vi "Module.Init Working Dirs.vi"(7 "Public Docs":bool, 8 "error in":errorcluster, 11 "App Name":string) -> (0 "error out":errorcluster, 3 "Working Dirs":T1)   [LabVIEW 2024, in "EQMF.lvlib" / "Module Utils.lvlib"]
uses:
  Module Utils.lvlib
  Module.Working Dirs.ctl
  <vilib>/Utility/sysdir.llb/System Directory Type.ctl
  <vilib>/Utility/config.llb/Read Key (Path).vi
  <vilib>/Utility/config.llb/NI_LVConfig.lvlib
  Files/File Utils.lvlib
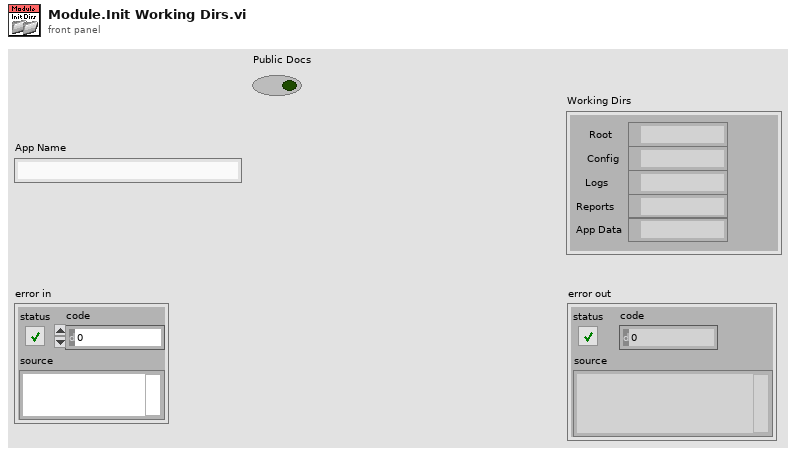
[diagram p1: front panel]
types:
  T1 = typedef "EQMF.lvlib/Module Utils.lvlib/Module.Working Dirs.ctl" = cluster{"Root":path, "Config":path, "Logs":path, "Reports":path, "App Data":path}
  T2 = enum32{"invalid app kind", "Development System", "Run Time System", "Student Edition", "Embedded LabVIEW", "Evaluation", "Custom"}
  T3 = cluster{"Working Dir":path, "Local Config File":path}
  T4 = typedef "NI_LVConfig.lvlib/Config Data RefNum.ctl" = refnum<k1>
  T5 = typedef "System Directory Type.ctl" = i32
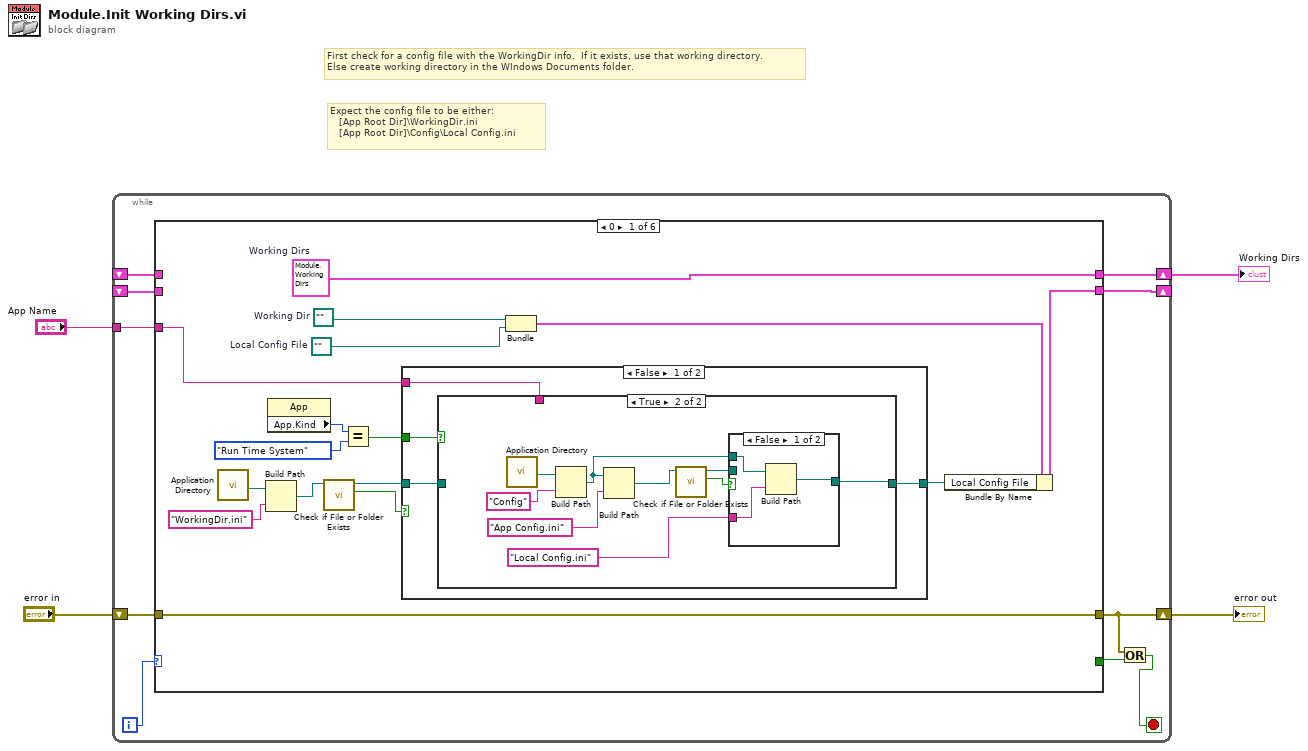
[diagram p0: block diagram]
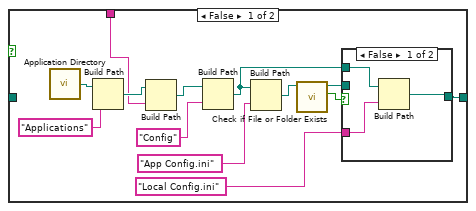
[diagram p2: hidden frame]
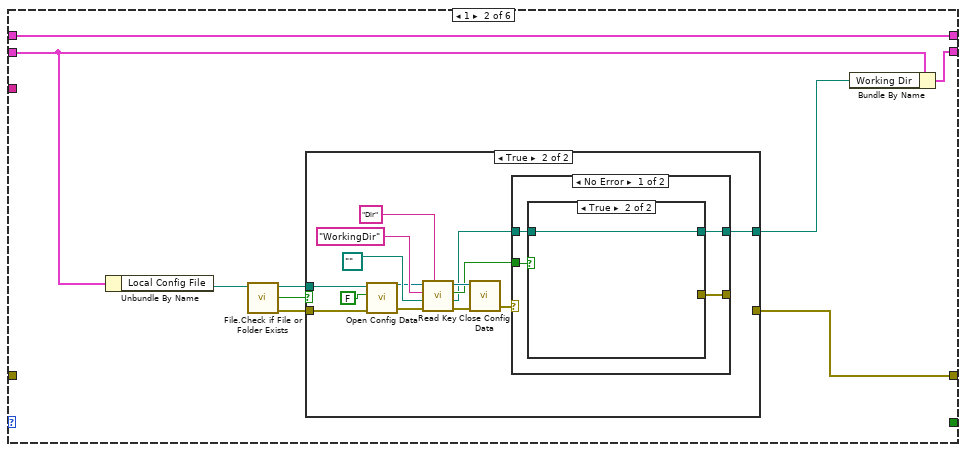
[diagram p6: hidden frame]
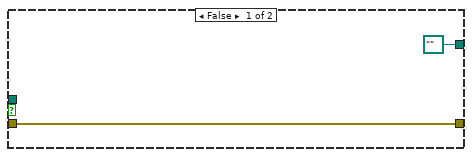
[diagram p7: hidden frame]
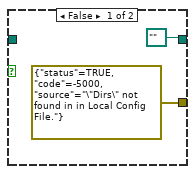
[diagram p8: hidden frame]
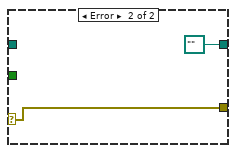
[diagram p9: hidden frame]
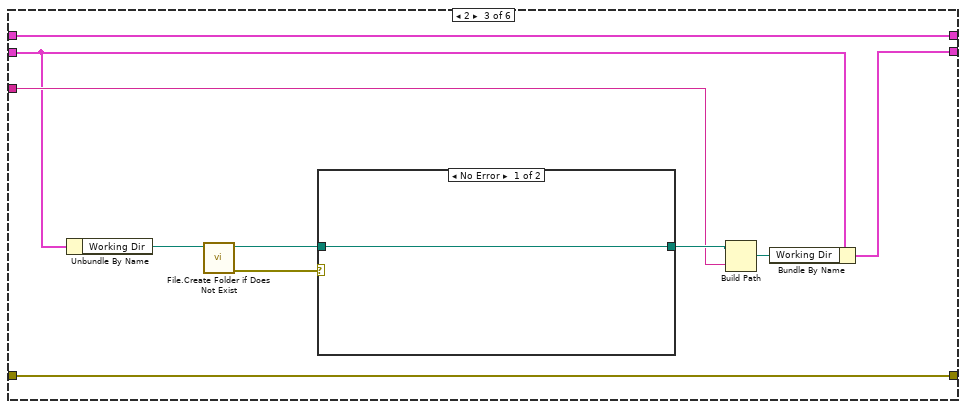
[diagram p10: hidden frame]
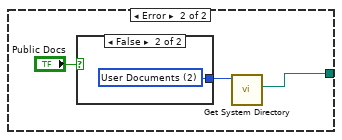
[diagram p11: hidden frame]
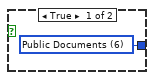
[diagram p12: hidden frame]
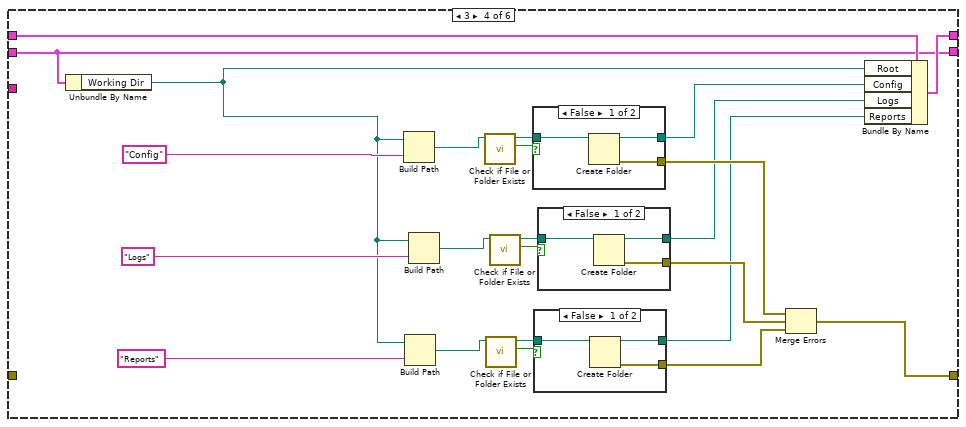
[diagram p13: hidden frame]
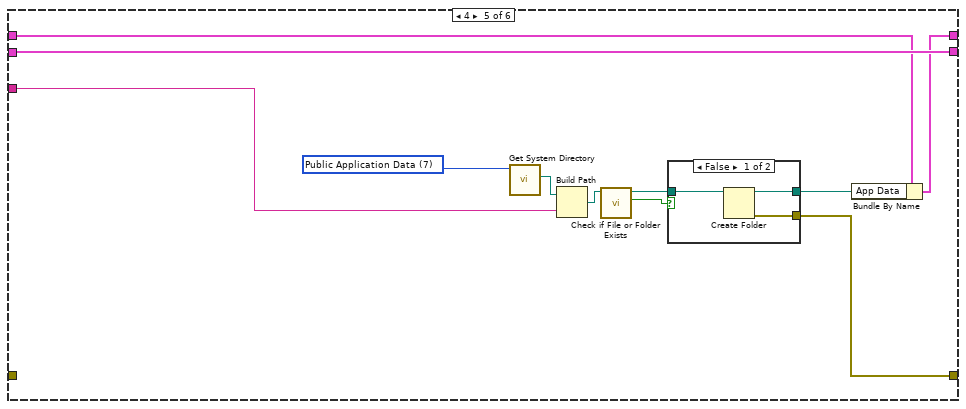
[diagram p17: hidden frame]
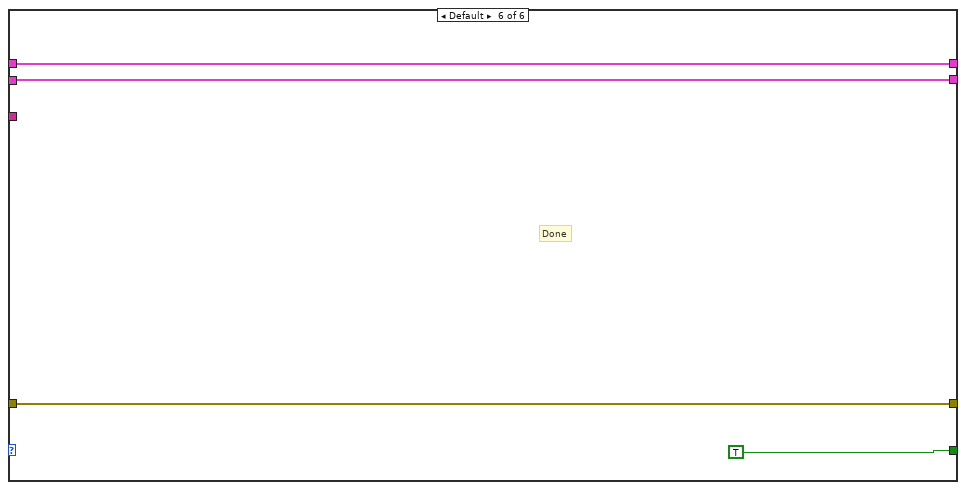
[diagram p19: hidden frame]
diagram:
  # "Expect the config file to be either:\n   [App Root Dir]\\WorkingDir.ini\n   [App Root Dir]\\Config\\Local Config.ini"
  # "First check for a config file with the WorkingDir info.  If it exists, use that working directory.\nElse create working directory in the WIndows Documents folder."
  n1 = while {
    shift-right: [w10] -> w3
    shift-left: "error in" -> [w13]
    shift-right: [w12] -> w1
    shift-left: _ -> [w7]
    tunnel: "App Name" -> [w8]
    shift-right: [w5] -> _
    shift-left: _ -> [w6]
    i -> [w14]
    stop <- w9 stop-if-true
    n2 = case shown="0" w14 {
      tunnel: [_ _ _ _ _ TRUE] -> w11
      tunnel: [w29 w70 w103 w118 w155 w168] -> w10
      tunnel: w13 -> [w29 _ w103 _ _ w168]
      tunnel: [w30 w71 w109 w137 w152 w167] -> w12
      tunnel: w8 -> [w16 _ w106 _ w156 _]
      tunnel: w7 -> [_ w71 w109 w138 w153 w167]
      tunnel: w6 -> [_ w68 w104 w116 w154 w166]
      tunnel: [w25 w69 w105 w116 w154 w166] -> w5
      frame 0 {
        w27 = path ""  # Local Config File
        w28 = path ""  # Working Dir
        w30 = T1 {"Root"=path "", "Config"=path "", "Logs"=path "", "Reports"=path "", "App Data"=path ""}  # Working Dirs
        n3 = call <vilib>:"Application Directory.vi"() -> ("Application Directory"=w21:path)
        n4 = Build Path(base path=w21, name or relative path="WorkingDir.ini") -> (appended path=w22:path)
        n5 = property class="App"() -> ("App.Kind"=w19:T2)  [unwired: 2 in, 2 out]
        n6 = call <vilib>:"Check if File or Folder Exists.vi"("path"=w22) -> ("file or folder exists?"=w24:bool, "dup path"=w23:path)  [unwired: 8 in, 1 out]
        n7 = Equal?(x=w19, y=T2."Run Time System" ("Application:Kind")) -> (x = y?=w20:bool)
        n8 = case shown="False" w24 {
          tunnel: w20 -> [w34 _]
          tunnel: w23 -> [w33 w65]
          tunnel: [w32 w65] -> w15
          tunnel: w16 -> [w31 _]
          frame False {
            n9 = case shown="True" w34 {
              tunnel: [w37 w53] -> w32
              tunnel: w33 -> [_ _]
              tunnel: w31 -> [w41 _]
              frame False {
                n10 = call <vilib>:"Application Directory.vi"() -> ("Application Directory"=w45:path)
                n11 = Build Path(base path=w45, name or relative path="Applications") -> (appended path=w46:path)
                n12 = Build Path(base path=w46, name or relative path=w41) -> (appended path=w47:path)
                n13 = Build Path(base path=w47, name or relative path="Config") -> (appended path=w35:path)
                n14 = Build Path(base path=w35, name or relative path="App Config.ini") -> (appended path=w40:path)
                n15 = call <vilib>:"Check if File or Folder Exists.vi"("path"=w40) -> ("file or folder exists?"=w39:bool, "dup path"=w38:path)  [unwired: 8 in, 1 out]
                n16 = case shown="False" w39 {
                  tunnel: w38 -> [_ w51]
                  tunnel: [w49 w51] -> w37
                  tunnel: "Local Config.ini" -> [w50 _]
                  tunnel: w35 -> [w48 _]
                  frame False {
                    n17 = Build Path(base path=w48, name or relative path=w50) -> (appended path=w49:path)
                  }
                  frame True {
                  }
                }
              }
              frame True {
                n18 = call <vilib>:"Application Directory.vi"() -> ("Application Directory"=w60:path)
                n19 = Build Path(base path=w60, name or relative path="Config") -> (appended path=w52:path)
                n20 = Build Path(base path=w52, name or relative path="App Config.ini") -> (appended path=w55:path)
                n21 = call <vilib>:"Check if File or Folder Exists.vi"("path"=w55) -> ("file or folder exists?"=w57:bool, "dup path"=w56:path)  [unwired: 8 in, 1 out]
                n22 = case shown="False" w57 {
                  tunnel: w56 -> [_ w64]
                  tunnel: [w62 w64] -> w53
                  tunnel: "Local Config.ini" -> [w63 _]
                  tunnel: w52 -> [w61 _]
                  frame False {
                    n23 = Build Path(base path=w61, name or relative path=w63) -> (appended path=w62:path)
                  }
                  frame True {
                  }
                }
              }
            }
          }
          frame True {
          }
        }
        n24 = Bundle("Working Dir"=w28, "Local Config File"=w27) -> (w26:T3)  [unwired: 1 in]
        n25 = Bundle By Name(cluster=w26, "Local Config File"=w15) -> (w25:T3)
      }
      frame 1 {
        n26 = Unbundle By Name(w68) -> ("Local Config File"=w67:path)
        n27 = call "File.Check if File or Folder Exists.vi"("Path"=w67) -> ("error out"=w73:errorcluster, "Exists"=w72:bool, "Dup Path"=w74:path)  [unwired: 6 in, 2 out]
        n28 = case shown="True" w72 {
          tunnel: w74 -> [_ w82]
          tunnel: w73 -> [w76 w81]
          tunnel: [w76 _] -> w70
          tunnel: [path "" w77] -> w66
          frame False {
          }
          frame True {
            n29 = call <vilib>:"Open Config Data.vi"("error in (no error)"=w81, "create file if necessary (T)"=FALSE, "configuration file path"=w82) -> ("error out"=w85:errorcluster, "refnum"=w86:T4)  [unwired: 6 in, 1 out]
            n30 = call-poly <vilib>:"Read Key.vi"("section"="Dir", "error in (no error)"=w85, "default value"=path "" ("Working Dir"), "key"="WorkingDir", "refnum"=w86) -> ("error out"=w84:errorcluster, "value"=w78:path, "found?"=w79:bool, "refnum out"=w83:T4)  [unwired: 3 in]
            n31 = call <vilib>:"Close Config Data.vi"("error in (no error)"=w84, "refnum"=w83) -> ("error out"=w80:errorcluster)  [unwired: 8 in, 1 out]
            n32 = case shown="No Error" w80 {
              selector: w80 -> [_ w99]
              tunnel: w79 -> [w94 _]
              tunnel: [w93 w99] -> _
              tunnel: w78 -> [w92 _]
              tunnel: [w91 path ""] -> w77
              frame No Error {
                n33 = case shown="True" w94 {
                  tunnel: [errorcluster {"status"=TRUE, "code"=-5000, "source"="\"Dirs\" not found in in Local Config File."} ("error constant") _] -> w93
                  tunnel: w92 -> [_ w97]
                  tunnel: [path "" w97] -> w91
                  frame False {
                  }
                  frame True {
                  }
                }
              }
              frame Error {
              }
            }
          }
        }
        n34 = Bundle By Name(cluster=w68, "Working Dir"=w66) -> (w69:T3)
      }
      frame 2 {
        n35 = Unbundle By Name(w104) -> ("Working Dir"=w102:path)
        n36 = call "File.Create Folder if Does Not Exist.vi"("Path"=w102) -> ("error out"=w101:errorcluster, "Dup Path"=w100:path)  [unwired: 8 in, 1 out]
        n37 = case shown="No Error" w101 {
          tunnel: w100 -> [w110 _]
          tunnel: [w110 w111] -> w107
          frame No Error {
          }
          frame Error {
            n38 = case shown="False" "Public Docs" {
              tunnel: [w114 w115] -> w112
              frame True {
                w114 = T5 6 items=["User Home"=0, "User Desktop"=1, "User Documents"=2, "User Application Data"=3, "User Preferences"=4, "User Temporary"=5, "Public Documents"=6, "Public Application Data"=7, "Public Preferences"=8, "Public Cache"=13, "System Core Libraries"=9, "System Installed Libraries"=10, "Application Files"=11, "Boot Volume Root"=12] ("system directory type")
              }
              frame False {
                w115 = T5 2 items=["User Home"=0, "User Desktop"=1, "User Documents"=2, "User Application Data"=3, "User Preferences"=4, "User Temporary"=5, "Public Documents"=6, "Public Application Data"=7, "Public Preferences"=8, "Public Cache"=13, "System Core Libraries"=9, "System Installed Libraries"=10, "Application Files"=11, "Boot Volume Root"=12] ("system directory type")
              }
            }
            n39 = call <vilib>:"Get System Directory.vi"("system directory type"=w112) -> ("system directory"=w111:path)  [unwired: 10 in]
          }
        }
        n40 = Build Path(base path=w107, name or relative path=w106) -> (appended path=w108:path)
        n41 = Bundle By Name(cluster=w104, "Working Dir"=w108) -> (w105:T3)
      }
      frame 3 {
        n42 = Unbundle By Name(w116) -> ("Working Dir"=w117:path)
        n43 = Build Path(base path=w117, name or relative path="Config") -> (appended path=w128:path)
        n44 = Build Path(base path=w117, name or relative path="Reports") -> (appended path=w126:path)
        n45 = Build Path(base path=w117, name or relative path="Logs") -> (appended path=w127:path)
        n46 = call <vilib>:"Check if File or Folder Exists.vi"("path"=w128) -> ("file or folder exists?"=w136:bool, "dup path"=w135:path)  [unwired: 8 in, 1 out]
        n47 = call <vilib>:"Check if File or Folder Exists.vi"("path"=w126) -> ("file or folder exists?"=w125:bool, "dup path"=w124:path)  [unwired: 8 in, 1 out]
        n48 = call <vilib>:"Check if File or Folder Exists.vi"("path"=w127) -> ("file or folder exists?"=w131:bool, "dup path"=w132:path)  [unwired: 8 in, 1 out]
        n49 = case shown="False" w136 {
          tunnel: [w149 _] -> w130
          tunnel: w135 -> [w148 w150]
          tunnel: [w147 w150] -> w122
          frame False {
            n50 = Create Folder(path (use dialog)=w148) -> (created path=w147:path, error out=w149:errorcluster)  [unwired: 2 in, 1 out]
          }
          frame True {
          }
        }
        n51 = case shown="False" w125 {
          tunnel: [w141 _] -> w119
          tunnel: w124 -> [w140 w142]
          tunnel: [w139 w142] -> w120
          frame False {
            n52 = Create Folder(path (use dialog)=w140) -> (created path=w139:path, error out=w141:errorcluster)  [unwired: 2 in, 1 out]
          }
          frame True {
          }
        }
        n53 = case shown="False" w131 {
          tunnel: [w145 _] -> w129
          tunnel: w132 -> [w144 w146]
          tunnel: [w143 w146] -> w121
          frame False {
            n54 = Create Folder(path (use dialog)=w144) -> (created path=w143:path, error out=w145:errorcluster)  [unwired: 2 in, 1 out]
          }
          frame True {
          }
        }
        n55 = Merge Errors(w130, w129, w119) -> (w118:errorcluster)
        n56 = Bundle By Name(cluster=w138, "Root"=w117, "Config"=w122, "Logs"=w121, "Reports"=w120) -> (w137:T1)
      }
      frame 4 {
        w160 = T5 7 items=["User Home"=0, "User Desktop"=1, "User Documents"=2, "User Application Data"=3, "User Preferences"=4, "User Temporary"=5, "Public Documents"=6, "Public Application Data"=7, "Public Preferences"=8, "Public Cache"=13, "System Core Libraries"=9, "System Installed Libraries"=10, "Application Files"=11, "Boot Volume Root"=12] ("system directory type")
        n57 = call <vilib>:"Get System Directory.vi"("system directory type"=w160) -> ("system directory"=w161:path)  [unwired: 10 in]
        n58 = Build Path(base path=w161, name or relative path=w156) -> (appended path=w159:path)
        n59 = call <vilib>:"Check if File or Folder Exists.vi"("path"=w159) -> ("file or folder exists?"=w158:bool, "dup path"=w157:path)  [unwired: 8 in, 1 out]
        n60 = case shown="False" w158 {
          tunnel: [w164 _] -> w155
          tunnel: w157 -> [w163 w165]
          tunnel: [w162 w165] -> w151
          frame False {
            n61 = Create Folder(path (use dialog)=w163) -> (created path=w162:path, error out=w164:errorcluster)  [unwired: 2 in, 1 out]
          }
          frame True {
          }
        }
        n62 = Bundle By Name(cluster=w153, "App Data"=w151) -> (w152:T1)
      }
      frame Default {
        # "Done"
      }
    }
    n63 = Or(x=w10, y=w11) -> (x .or. y?=w9:bool)
  }
  "Working Dirs" <- w1
  "error out" <- w3
